vi "Vbias Lookup Table.vi"() -> (2 "ROUT<7:5>":u8[](array[numeric])=[7, 6, 5, 4, 0, 1, 2, 3], 3 "VB(V)":dbl[](array[numeric])=[14.1, 12.6, 13.1, 13.6, 12.1, 11.6, 11.1, 14.1])   [LabVIEW 2020]
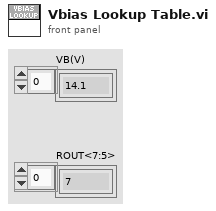
[diagram p1: front panel]
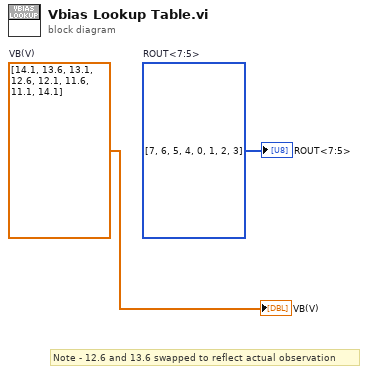
[diagram p0: block diagram]
diagram:
  w2 = dbl[] [14.1, 13.6, 13.1, 12.6, 12.1, 11.6, 11.1, 14.1]  # VB(V)
  w1 = u8[] [7, 6, 5, 4, 0, 1, 2, 3]  # ROUT<7:5>
  # "Note - 12.6 and 13.6 swapped to reflect actual observation"
  "VB(V)" <- w2
  "ROUT<7:5>" <- w1
